vi "Check Variant Type.vi"(8 "error in (no error)":errorcluster, 10 "Variant":variant, 11 "Value Type in":refnum<class "Value Type.lvclass">) -> (0 "error out":errorcluster, 3 "Value Type out":refnum<class "Value Type.lvclass">)   [LabVIEW 2020, in "Composed Columns.lvlib" / "Value Type.lvclass"]
uses:
  Value Type.lvclass
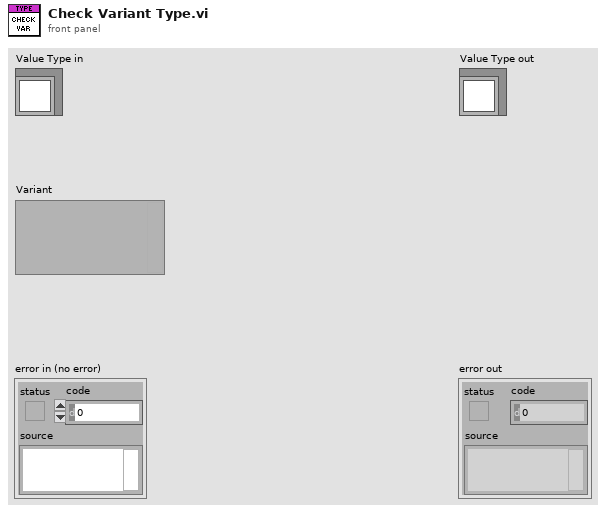
[diagram p1: front panel]
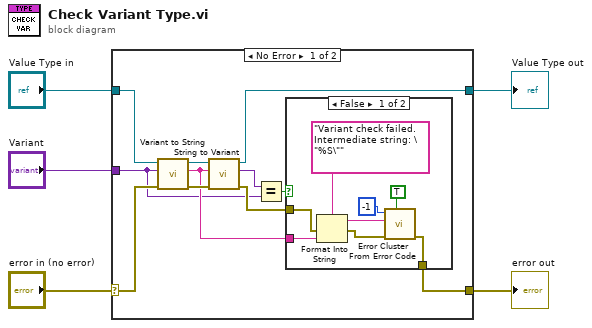
[diagram p0: block diagram]
diagram:
  n1 = case shown="No Error" "error in (no error)" {
    selector: "error in (no error)" -> [w13 w27]
    tunnel: [w11 w27] -> w4
    tunnel: [w14 w26] -> w2
    tunnel: "Value Type in" -> [w16 w26]
    tunnel: "Variant" -> [w6 _]
    frame No Error {
      n2 = call-dynamic "Variant to String.vi"("error in (no error)"=w13, "Variant"=w6, "Value Type in"=w16) -> ("error out"=w12:errorcluster, "String"=w10:string, "Value Type out"=w15:refnum<class "Value Type.lvclass">)  [unwired: 6 in]
      n3 = call-dynamic "String to Variant.vi"("error in (no error)"=w12, "String"=w10, "Value Type in"=w15) -> ("error out"=w8:errorcluster, "Variant"=w7:variant, "Value Type out"=w14:refnum<class "Value Type.lvclass">)  [unwired: 6 in]
      n4 = Equal?(x=w7, y=w6) -> (x = y?=w9:bool)
      n5 = case shown="False" w9 {
        tunnel: w10 -> [w23 _]
        tunnel: [w20 w25] -> w11
        tunnel: w8 -> [w18 w25]
        frame False {
          n6 = Format Into String(format string="Variant check failed. Intermediate string: \"%S\"", error in=w18, w23) -> (resulting string=w21:string, error out=w17:errorcluster)  [unwired: 1 in]
          n7 = call <vilib>:"Error Cluster From Error Code.vi"("show call chain? (False)"=TRUE, "error in (no error)"=w17, "error message (\"\")"=w21, "error code (0)"=-1) -> ("error out"=w20:errorcluster)  [unwired: 5 in]
        }
        frame True {
        }
      }
    }
    frame Error {
    }
  }
  "error out" <- w4
  "Value Type out" <- w2
